vi "z hello locators.vi"(8 "error in (no error)":errorcluster, 10 "locators_out":cluster{}, 11 "this_":cluster{}) -> (0 "error out":errorcluster, 2 "locators_out out":cluster{})   [LabVIEW 2021, in "zenohc.lvlib"]
doc: "void z_hello_locators(const struct z_loaned_hello_t *this_,\n struct z_owned_string_array_t *locators_out);"
uses:
  zenohc.lvlib
  zenohc.dll
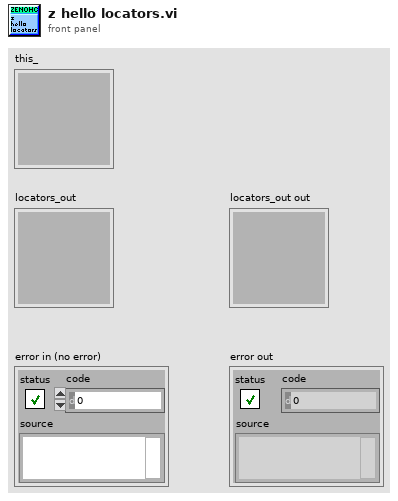
[diagram p1: front panel]
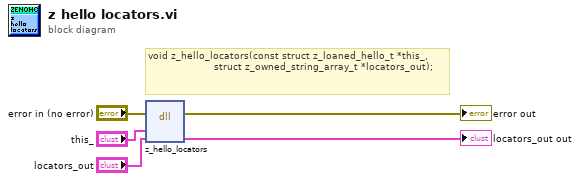
[diagram p0: block diagram]
diagram:
  # "void z_hello_locators(const struct z_loaned_hello_t *this_,\n                      struct z_owned_string_array_t *locators_out);"
  n1 = dll-call lib="D:/dev/zenoh_labview/zenohc/zenohc.*" fn="z_hello_locators"(error in="error in (no error)", "this_"="this_", "locators_out"="locators_out") -> (error out=→"error out":errorcluster, "locators_out"=→"locators_out out":cluster{})  [unwired: 4 in, 1 out]
